vi "coincidence stats.vi"(8 "error in":errorcluster, 10 "Action":enum16{"Insert", "Get", "Initiate"}(ring), 11 "New data":T2(array[cluster])) -> (0 "error out":errorcluster, 2 "Sum":i32[][](array[numeric]), 3 "Coinc stats":T1={"Numofpoints"=10000, "Current index"=0, "Max index"=0, "Data"=[{"initialized array"=[[0, 0, 0, 0, 0, 0, 0, 0, 0, 0, 0, 0], [0, 0, 0, 0, 0, 0, 0, 0, 0, 0, 0, 0], [0, 0, 0, 0, 0, 0, 0, 0, 0, 0, 0, 0], [0, 0, 0, 0, 0, 0, 0, 0, 0, 0, 0, 0], [0, 0, 0, 0, 0, 0, 0, 0, 0, 0, 0, 0], [0, 0, 0, 0, 0, 0, 0, 0, 0, 0, 0, 0], [0, 0, 0, 0, 0, 0, 0, 0, 0, 0, 0, 0], [0, 0, 0, 0, 0, 0, 0, 0, 0, 0, 0, 0], [0, 0, 0, 0, 0, 0, 0, 0, 0, 0, 0, 0], [0, 0, 0, 0, 0, 0, 0, 0, 0, 0, 0, 0], [0, 0, 0, 0, 0, 0, 0, 0, 0, 0, 0, 0], [0, 0, 0, 0, 0, 0, 0, 0, 0, 0, 0, 0]], "Timestamp"=timestamp(0 s since 1904-01-01)}], "Filled"=FALSE})   [LabVIEW 2016]
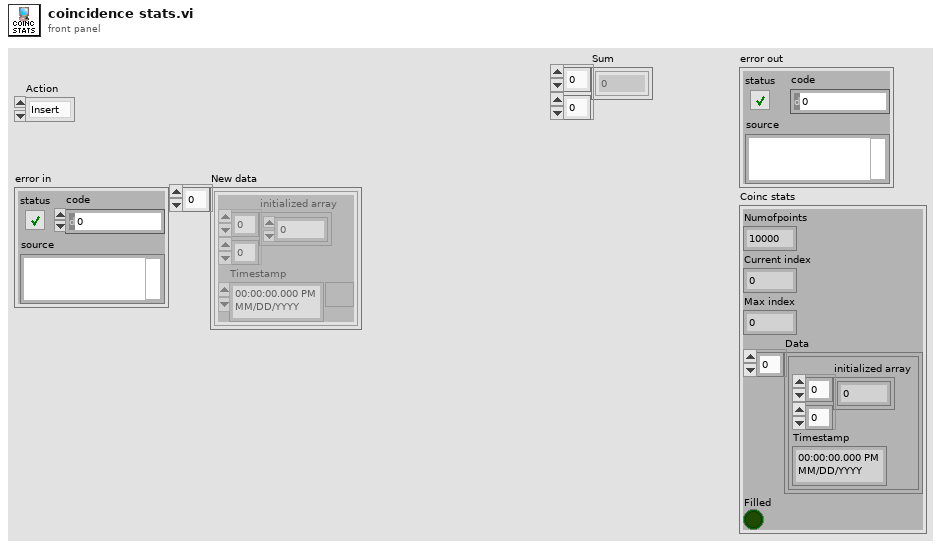
[diagram p1: front panel]
types:
  T1 = cluster{"Numofpoints":i32, "Current index":i32, "Max index":i32, "Data":cluster{"initialized array":i32[][], "Timestamp":timestamp}[], "Filled":bool}
  T2 = cluster{"initialized array":i32[][], "Timestamp":timestamp}[]
  T3 = cluster{"initialized array":i16[][], "Timestamp":timestamp}[]
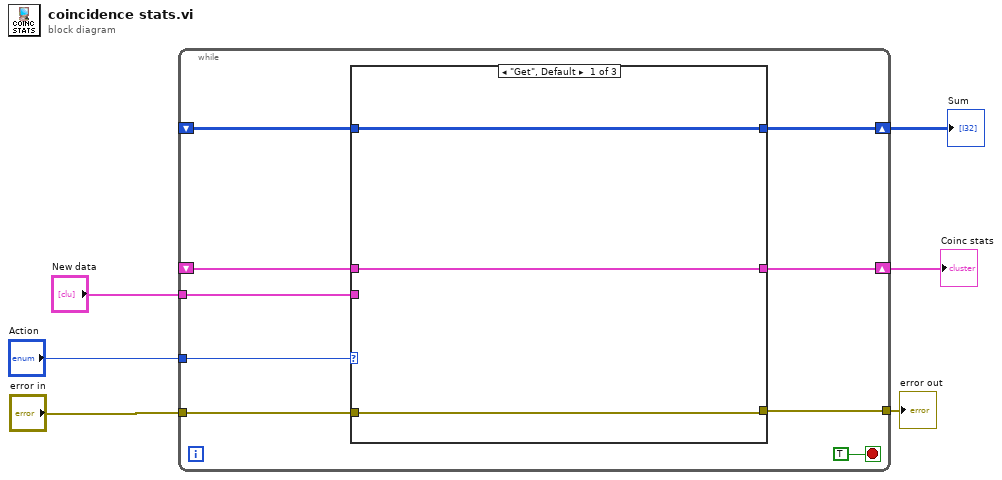
[diagram p0: block diagram]
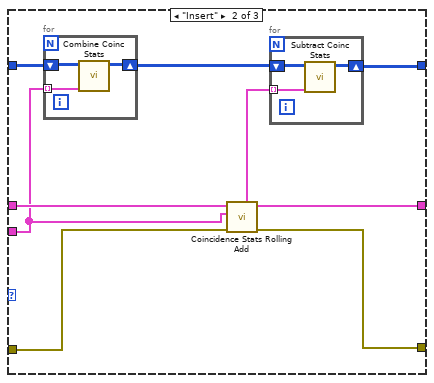
[diagram p2: hidden frame]
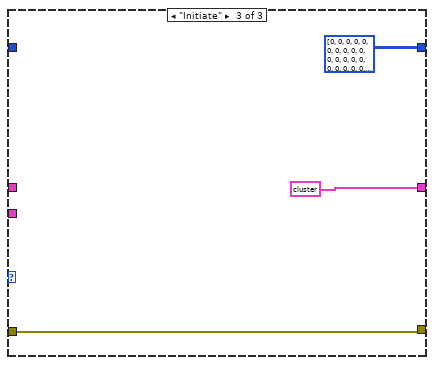
[diagram p3: hidden frame]
diagram:
  n1 = while {
    shift-right: [w15] -> w1
    shift-left: _ -> [w14]
    tunnel: "Action" -> [w13]
    tunnel: "error in" -> [w12]
    tunnel: [w11] -> w3
    tunnel: "New data" -> [w10]
    shift-right: [w8] -> w2
    shift-left: _ -> [w7]
    stop <- TRUE stop-if-true
    n2 = case shown="\"Get\", Default" w13 {
      tunnel: [w18 w26 T1 {"Numofpoints"=0, "Current index"=0, "Max index"=9999, "Data"=array[10000 elements], "Filled"=FALSE} ("Rolling array in")] -> w15
      tunnel: w14 -> [w18 w27 _]
      tunnel: w12 -> [w17 w25 w35]
      tunnel: [w17 w24 w35] -> w11
      tunnel: w10 -> [_ w23 _]
      tunnel: [w16 w20 i32[][] [[0, 0, 0, 0, 0, 0, 0, 0, 0, 0, 0, 0], [0, 0, 0, 0, 0, 0, 0, 0, 0, 0, 0, 0], [0, 0, 0, 0, 0, 0, 0, 0, 0, 0, 0, 0], [0, 0, 0, 0, 0, 0, 0, 0, 0, 0, 0, 0], [0, 0, 0, 0, 0, 0, 0, 0, 0, 0, 0, 0], [0, 0, 0, 0, 0, 0, 0, 0, 0, 0, 0, 0], [0, 0, 0, 0, 0, 0, 0, 0, 0, 0, 0, 0], [0, 0, 0, 0, 0, 0, 0, 0, 0, 0, 0, 0], [0, 0, 0, 0, 0, 0, 0, 0, 0, 0, 0, 0], [0, 0, 0, 0, 0, 0, 0, 0, 0, 0, 0, 0], [0, 0, 0, 0, 0, 0, 0, 0, 0, 0, 0, 0], [0, 0, 0, 0, 0, 0, 0, 0, 0, 0, 0, 0]] ("initialized array")] -> w8
      tunnel: w7 -> [w16 w22 _]
      frame "Get", Default {
      }
      frame "Insert" {
        n3 = for {
          tunnel: w23 -> [w31] mode=indexing
          shift-right: [w33] -> w21
          shift-left: w22 -> [w32]
          n4 = call "Combine Coinc Stats.vi"("New statistics"=w31, "Existing statistics"=w32) -> ("Output"=w33:i32[][])  [unwired: 9 in]
        }
        n5 = call "Coincidence Stats Rolling Add.vi"("error in (no error)"=w25, "New data"=w23, "Rolling array in"=w27) -> ("error out"=w24:errorcluster, "Rolling array out"=w26:T1, "Removed elements"=w19:T3)  [unwired: 5 in, 1 out]
        n6 = for {
          tunnel: w19 -> [w28] mode=indexing
          shift-right: [w30] -> w20
          shift-left: w21 -> [w29]
          n7 = call "Subtract Coinc Stats.vi"("Statistics to remove"=w28, "Existing statistics"=w29) -> ("Output"=w30:i32[][])  [unwired: 9 in]
        }
      }
      frame "Initiate" {
      }
    }
  }
  "error out" <- w3
  "Sum" <- w2
  "Coinc stats" <- w1
